vi "AIScaleAndLimit.vi"(0 "UnscaledAI":i16[](array[numeric])=[0, 0, 0, 0, 0, 0, 0, 0, 0, 0, 0, 0, 0, 0, 0, 0], 1 "RawAIConfig":T1={"AI16Limits"={"LimitsEnabled"=0, "UnscaledHighLimit"=[0, 0, 0, 0, 0, 0, 0, 0, 0, 0, 0, 0, 0, 0, 0, 0], "UnscaledLowLimit"=[0, 0, 0, 0, 0, 0, 0, 0, 0, 0, 0, 0, 0, 0, 0, 0]}, "AI16ScaleConfig"={"B"=[0, 0, 0, 0, 0, 0, 0, 0, 0, 0, 0, 0, 0, 0, 0, 0], "M"=[0.0, 0.0, 0.0, 0.0, 0.0, 0.0, 0.0, 0.0, 0.0, 0.0, 0.0, 0.0, 0.0, 0.0, 0.0, 0.0]}} {"AI16Limits"."LimitsEnabled" format="%.0x"}, 7 "ClearFaults":bool, 9 "input valid":bool=TRUE) -> (4 "ScaledAI":sgl[](array[numeric]), 8 "AILimits":bool, 10 "ready for input":bool, 13 "AILimitHigh":u16 format="%.0x", 14 "ALimitLow":u16 format="%.0x", 15 "output valid":bool)   [LabVIEW 2015, in "ScaleAndLimit.lvlib"]
uses:
  ScaleAndLimit.lvlib
  ScaleAndLimitAI16Config.ctl
  AI16LimitsConfig.ctl
  AI16ScaleConfig.ctl
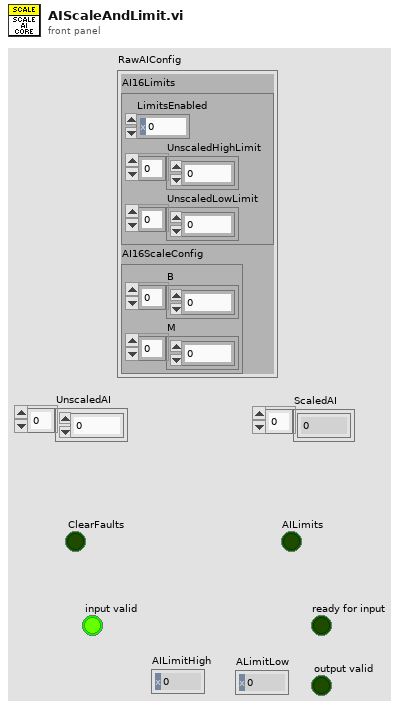
[diagram p1: front panel]
types:
  T1 = typedef "ScaleAndLimit.lvlib/ScaleAndLimitAI16Config.ctl" = cluster{"AI16Limits":T2, "AI16ScaleConfig":T3}
  T2 = typedef "ScaleAndLimit.lvlib/AI16LimitsConfig.ctl" = cluster{"LimitsEnabled":u16, "UnscaledHighLimit":i16[], "UnscaledLowLimit":i16[]}
  T3 = typedef "ScaleAndLimit.lvlib/AI16ScaleConfig.ctl" = cluster{"B":i16[], "M":sgl[]}
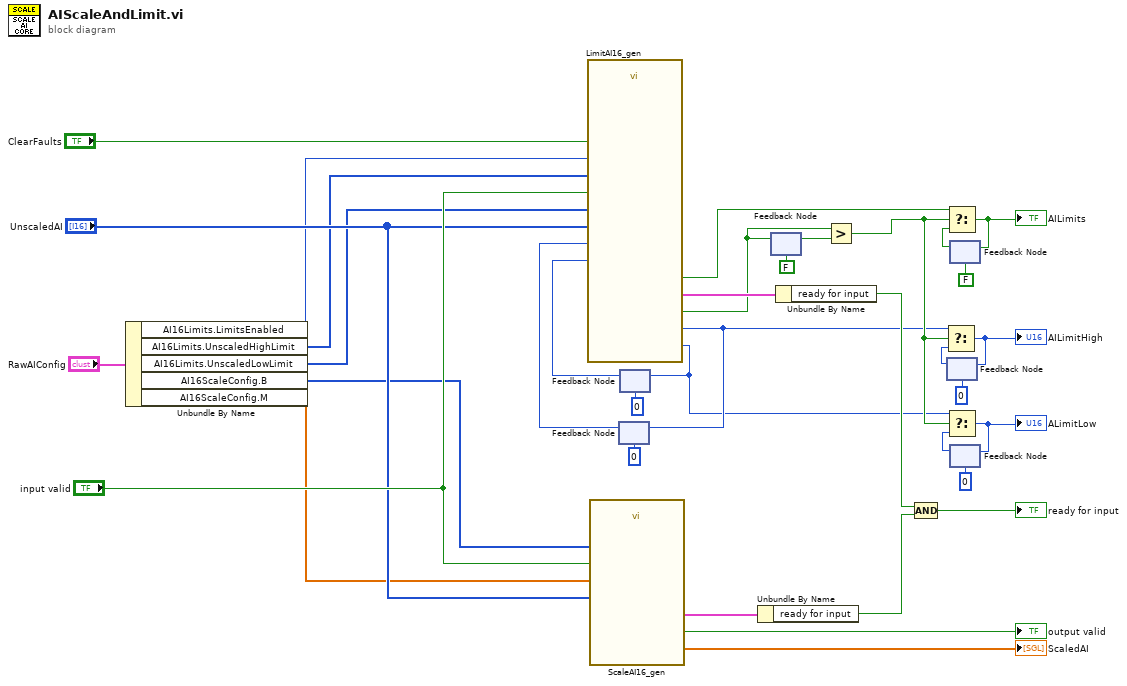
[diagram p0: block diagram]
diagram:
  n1 = Unbundle By Name("RawAIConfig") -> ("AI16Limits.LimitsEnabled"=w5:u16, "AI16Limits.UnscaledHighLimit"=w4:i16[], "AI16Limits.UnscaledLowLimit"=w3:i16[], "AI16ScaleConfig.B"=w2:i16[], "AI16ScaleConfig.M"=w1:sgl[])
  n2 = call "ScaleAI16_gen.vi"("M"=w1, "B"=w2, "RawAI"="UnscaledAI", "input valid"="input valid") -> ("ScaledAI"=→"ScaledAI":sgl[], "output valid"=→"output valid":bool, "feedback signals"=w29:cluster{"ready for input":bool})  [unwired: 9 in]
  n3 = feedback #1(u16 0 ("RawAIFaultHighOut")) -> (w34:u16)
  n4 = feedback #2(u16 0 ("RawAIFaultLowOut")) -> (w33:u16)
  n5 = call "LimitAI16_gen.vi"("ClearLimit"="ClearFaults", "HighLimit"=w4, "UnscaledAI"="UnscaledAI", "UnscaledLimitLowIn"=w33, "UnscaledLimitHighIn"=w34, "input valid"="input valid", "LowLimit"=w3, "LimitiEnabled"=w5) -> ("UnscaledLimitLowOut"=w13:u16, "UnscaledLimitHighOut"=w16:u16, "LimitReached"=w21:bool, "output valid"=w22:bool, "feedback signals"=w30:cluster{"ready for input":bool})  [unwired: 3 in]
  n6 = feedback-in #1(w16) -> ()
  n7 = feedback-in #2(w13) -> ()
  n8 = Unbundle By Name(w29) -> ("ready for input"=w27:bool)
  n9 = feedback-in #3(w22) -> ()
  n10 = feedback #3(FALSE ("faulted")) -> (w23:bool)
  n11 = Unbundle By Name(w30) -> ("ready for input"=w28:bool)
  n12 = Greater?(x=w22, y=w23) -> (0:w17:bool)
  n13 = Compound Arithmetic op=AND(w28, w27) -> (→"ready for input":bool)
  n14 = feedback #4(u16 0 ("RawAIFaultHighOut")) -> (w14:u16)
  n15 = Select(t=w16, s=w17, f=w14) -> (s? t:f=w15:u16)
  "AILimitHigh" <- w15
  n16 = feedback-in #4(w15) -> ()
  n17 = feedback #5(FALSE ("faulted")) -> (w19:bool)
  n18 = Select(t=w21, s=w17, f=w19) -> (s? t:f=w20:bool)
  "AILimits" <- w20
  n19 = feedback-in #5(w20) -> ()
  n20 = feedback #6(u16 0 ("RawAIFaultLowOut")) -> (w11:u16)
  n21 = Select(t=w13, s=w17, f=w11) -> (s? t:f=w12:u16)
  "ALimitLow" <- w12
  n22 = feedback-in #6(w12) -> ()
